vi "Test tiroir de com T-COM J1.vi"() -> ()   [LabVIEW 2020]
uses:
  <vilib>/MakerHub/LINX/Public/Peripherals/Analog/Analog Read N Chans.vi
  <vilib>/MakerHub/LINX/Public/Peripherals/Digital/Digital Write N Chans.vi
  <vilib>/MakerHub/LINX/Private/Local IO/LinxAnalogRead.vi
  <vilib>/MakerHub/LINX/Public/Utilities/Check Channel.vi
  <vilib>/MakerHub/LINX/Private/Local IO/LinxDigitalWrite.vi
  <vilib>/MakerHub/LINX/Public/Utilities/Open Serial.vi
  <vilib>/MakerHub/LINX/Private/Utilties/Generate Error.vi
  <vilib>/MakerHub/LINX/LMH-LINX.lvlib
panel:
  out "Voltages":dbl[](array[numeric])
  out "Device Name":string
  out "Error Out":errorcluster
  in  "Serial Port":refnum<visa-resource-name>="COM51"
  out "Numeric":i32
  in  "Values":bool[](array[boolean])=[FALSE, FALSE, FALSE, FALSE, FALSE]
  in  "stop":bool
  # "NC\n\nBATT\n\n\nVEH\n\n\nAUTO"
  # "R1:  CH1 24V                                   \n\nR2:  CH2  WAKEUP\n\nR3: 5V sur D3 \n\nR4:  Ne pas utiliser"
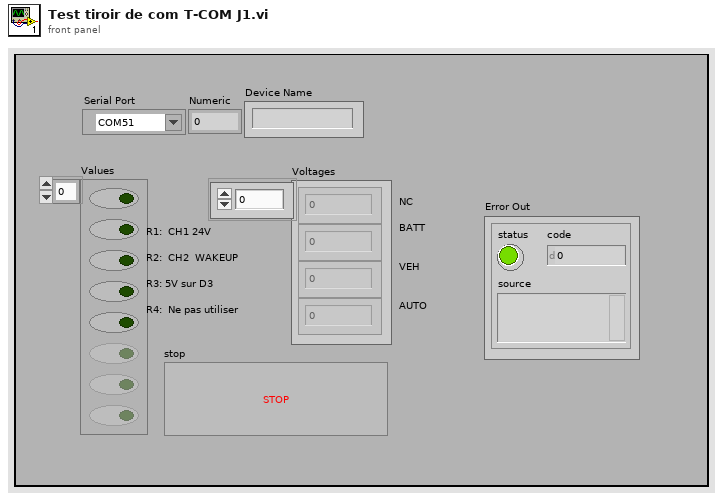
[diagram p1: front panel]
types:
  T1 = typedef "LMH-LINX.lvlib/LINX Ref.ctl" = cluster{"IO":T2, "Interface":T3, "LINX Device Config":T4}
  T2 = typedef "LMH-LINX.lvlib/Platform.ctl" = enum16{"Remote", "Local"}
  T3 = typedef "LMH-LINX.lvlib/Interface.ctl" = enum16{"Serial", "TCP"}
  T4 = typedef "LMH-LINX.lvlib/Device.lvlib/LINX Device Config.ctl" = cluster{"Interface":T3, "COM Port":refnum<visa-resource-name>, "TCP Configuration":T5, "Device Family":u8, "Device ID":u8, "Device Name":string, "TCP Ref":refnum<k5>, "Channels":T6}
  T5 = typedef "LMH-LINX.lvlib/Device.lvlib/TCP Config.ctl" = cluster{"IP Address":string, "Port":u16}
  T6 = typedef "LMH-LINX.lvlib/Channels.ctl" = cluster{"DI":u8[], "DO":u8[], "AI":u8[], "AO":u8[], "PWM":u8[], "QE":u8[], "UART":u8[], "I2C 2":u8[], "SPI":u8[], "CAN":u8[], "Servo":u8[], "AI Ref (V)":dbl, "AI Resolution (Bits)":u8, "AO Ref (V)":dbl, "AO Resolution (Bits)":u8}
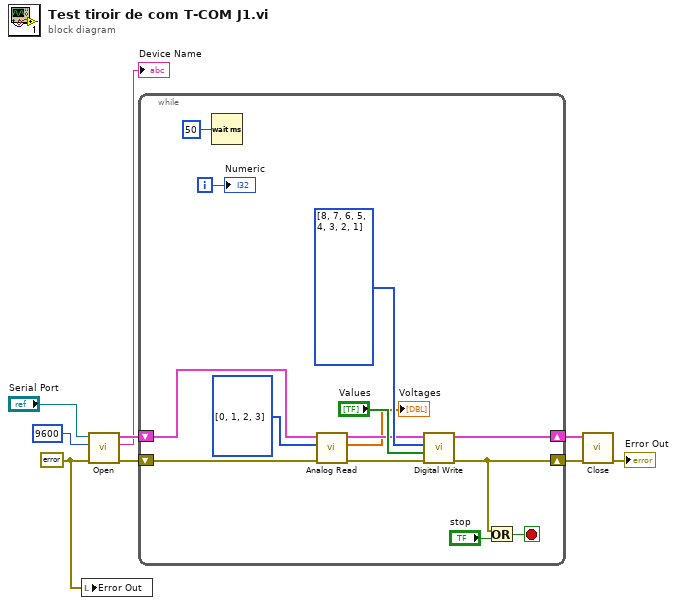
[diagram p0: block diagram]
diagram:
  w2 = errorcluster {"status"=FALSE, "code"=0, "source"=""} ("Error Out")
  n1 = local write "Error Out"(w2) -> ()
  n2 = call-poly <vilib>:"Open.vi"("Error In"=w2, "Baud Rate Override"=u32 9600, "Serial Port"="Serial Port") -> ("Error Out"=w3:errorcluster, "Device Name"=→"Device Name":string, "LINX Resource"=w6:T1)  [unwired: 6 in]
  n3 = while {
    shift-right: [w16] -> w7
    shift-left: w3 -> [w14]
    shift-right: [w17] -> w5
    shift-left: w6 -> [w13]
    i -> [w22]
    stop <- w18 stop-if-true
    n4 = Wait (ms)(milliseconds to wait=u32 50) -> ()  [unwired: 1 out]
    n5 = call-poly <vilib>:"Analog Read.vi"("Error In"=w14, "AI Channel(s)"=u8[] [0, 1, 2, 3] ("DI Channels"), "LINX Resource"=w13) -> ("Error Out"=w15:errorcluster, "Voltages"=→"Voltages":dbl[], "LINX Resource"=w12:T1)  [unwired: 5 in, 1 out]
    n6 = call-poly <vilib>:"Digital Write.vi"("Error In"=w15, "Values"="Values", "DO Channels"=u8[] [8, 7, 6, 5, 4, 3, 2, 1], "LINX Resource"=w12) -> ("Error Out"=w16:errorcluster, "LINX Resource"=w17:T1)  [unwired: 6 in]
    n7 = Or(x=w16, y="stop") -> (x .or. y?=w18:bool)
    "Numeric" <- w22
  }
  n8 = call <vilib>:"Close.vi"("Error In"=w7, "LINX Resource"=w5) -> ("Error Out"=→"Error Out":errorcluster)  [unwired: 9 in]
